vi "InMemo.vi"   [LabVIEW 2014]
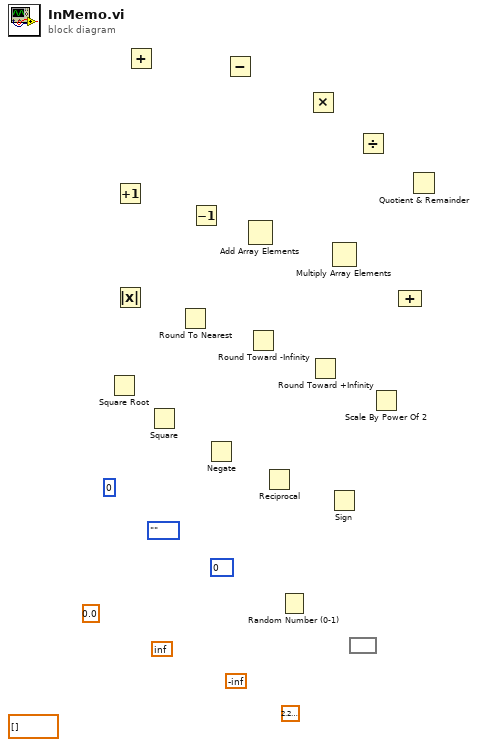
[diagram p0: block diagram]
diagram:
  (unwired) dbl[] []
  (unwired) 2.220446049250313e-16 ("Machine Epsilon")
  (unwired) -inf ("Negative Infinity")
  (unwired) inf ("Positive Infinity")
  (unwired) 0.0
  (unwired) u16 0 items=[""]
  (unwired) enum16{""}.""
  (unwired) 0
  n1 = Square Root() -> ()  [unwired: 1 in, 1 out]
  n2 = Increment() -> ()  [unwired: 1 in, 1 out]
  n3 = Absolute Value() -> ()  [unwired: 1 in, 1 out]
  n4 = Add() -> ()  [unwired: 2 in, 1 out]
  n5 = Square() -> ()  [unwired: 1 in, 1 out]
  n6 = Round To Nearest() -> ()  [unwired: 1 in, 1 out]
  n7 = Decrement() -> ()  [unwired: 1 in, 1 out]
  n8 = Negate() -> ()  [unwired: 1 in, 1 out]
  n9 = Subtract() -> ()  [unwired: 2 in, 1 out]
  n10 = Add Array Elements() -> ()  [unwired: 1 in, 1 out]
  n11 = Round Toward -Infinity() -> ()  [unwired: 1 in, 1 out]
  n12 = Reciprocal() -> ()  [unwired: 1 in, 1 out]
  n13 = Random Number (0-1)() -> ()  [unwired: 1 out]
  n14 = Multiply() -> ()  [unwired: 2 in, 1 out]
  n15 = Round Toward +Infinity() -> ()  [unwired: 1 in, 1 out]
  n16 = Multiply Array Elements() -> ()  [unwired: 1 in, 1 out]
  n17 = Sign() -> ()  [unwired: 1 in, 1 out]
  n18 = expression code=""() -> ()  [unwired: 1 in, 1 out]
  n19 = Divide() -> ()  [unwired: 2 in, 1 out]
  n20 = Scale By Power Of 2() -> ()  [unwired: 2 in, 1 out]
  n21 = Compound Arithmetic op=ADD() -> ()  [unwired: 2 in, 1 out]
  n22 = Quotient & Remainder() -> ()  [unwired: 2 in, 2 out]
